vi "Initialize.vi"(8 "error in (no error)":errorcluster, 9 "Project Path":path, 10 "New ID":bool, 11 "Step in":refnum<class "Step.lvclass">) -> (0 "error out":errorcluster, 3 "Step out":refnum<class "Step.lvclass">)   [LabVIEW 2015, in "Step.lvclass"]
uses:
  Step.lvclass
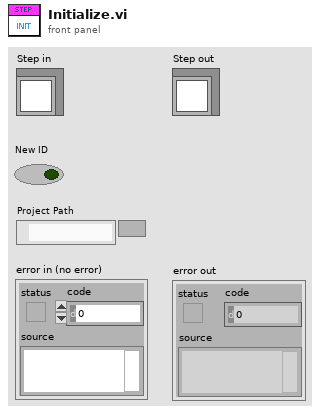
[diagram p1: front panel]
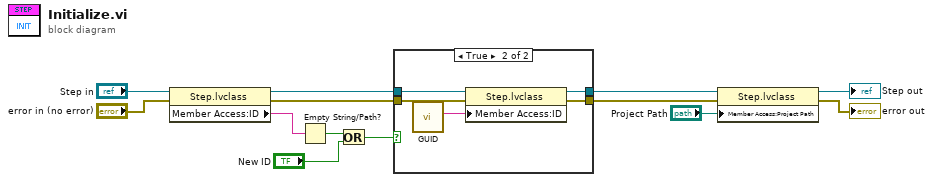
[diagram p0: block diagram]
diagram:
  n1 = property class="Step.lvclass"(reference="Step in", error in="error in (no error)") -> (reference out=w13:refnum<class "Step.lvclass">, error out=w12:errorcluster, "Member Access:ID"=w11:string)
  n2 = Empty String/Path?(string/path=w11) -> (empty?=w5:bool)
  n3 = Or(x=w5, y="New ID") -> (x .or. y?=w3:bool)
  n4 = case shown="True" w3 {
    tunnel: [w14 w19] -> w2
    tunnel: [w15 w18] -> w8
    tunnel: w13 -> [w15 w17]
    tunnel: w12 -> [w14 w16]
    frame False {
    }
    frame True {
      n5 = call "GUID.vi"() -> ("GUID"=w20:string)  [unwired: 10 in, 1 out]
      n6 = property class="Step.lvclass"(reference=w17, error in=w16, "Member Access:ID"=w20) -> (reference out=w18:refnum<class "Step.lvclass">, error out=w19:errorcluster)
    }
  }
  n7 = property class="Step.lvclass"(reference=w8, error in=w2, "Member Access:Project Path"="Project Path") -> (reference out=→"Step out":refnum<class "Step.lvclass">, error out=→"error out":errorcluster)
